vi "In Place Data Modification.vi"() -> ()   [LabVIEW 2019, in "Tree Map.lvlib"]
doc: "<b>Author:</b> Piotr Kruczkowski <PrimaryKey>\n<b>License:</b> NewBSD\n\nCopyright (c) 2019, National Instruments\nAll rights reserved.\n\nRedistribution and use in source and binary forms, with or without\nmodification, are permitted provided that the following conditions are met:\n1. Redistributions of source code must retain the above copyright\n notice, this list of conditions and the following disclaimer.\n2. Redistributions in binary form must reproduce the above copyright\n notice, this list of conditions and the following disclaimer in the\n documentation and/or other materials provided with the distribution.\n3. Neither the name of National Instruments nor the\n names of its contributors may be used to endorse or promote products\n derived from this software without specific prior written permission.\n\nTHIS SOFTWARE IS PROVIDED BY National Instruments ''AS IS'' AND ANY\nEXPRESS OR IMPLIED WARRANTIES, INCLUDING, BUT NOT LIMITED TO, THE IMPLIED\nWARRANTIES OF MERCHANTABILITY AND FITNESS FOR A PARTICULAR PURPOSE ARE\nDISCLAIMED. IN NO EVENT SHALL National Instruments BE LIABLE FOR ANY\nDIRECT, INDIRECT, INCIDENTAL, SPECIAL, EXEMPLARY, OR CONSEQUENTIAL DAMAGES\n(INCLUDING, BUT NOT LIMITED TO, PROCUREMENT OF SUBSTITUTE GOODS OR SERVICES;\nLOSS OF USE, DATA, OR PROFITS; OR BUSINESS INTERRUPTION) HOWEVER CAUSED AND\nON ANY THEORY OF LIABILITY, WHETHER IN CONTRACT, STRICT LIABILITY, OR TORT\n(INCLUDING NEGLIGENCE OR OTHERWISE) ARISING IN ANY WAY OUT OF THE USE OF THIS\nSOFTWARE, EVEN IF ADVISED OF THE POSSIBILITY OF SUCH DAMAGE."
uses:
  Tree Map.lvlib
panel:
  out "Pretty XML":string="<System>\n    <Configuration>\n        <Frequency>50.00</Frequency>\n    </Configuration>\n</System>"
  out "Frequency Node Path":string="\\System\\Configuration\\Frequency"
  in  "New Frequency":dbl=50.0 format="%#_13g"
  in  "Frequency":dbl=123.0 format="%#_13g"
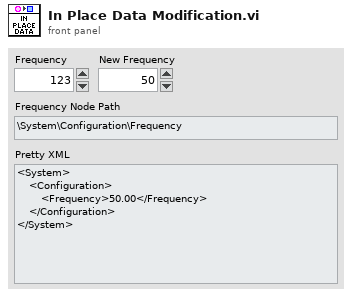
[diagram p1: front panel]
types:
  T1 = typedef "Tree Map.lvlib/Tree Map Data.ctl" = map{string, cluster{"Child Paths Set":set{string}, "Name":string, "Data":string, "Attributes":map{string, string}}}
  T2 = cluster{"Child Paths Set":set{string}, "Name":string, "Data":string, "Attributes":map{string, string}}
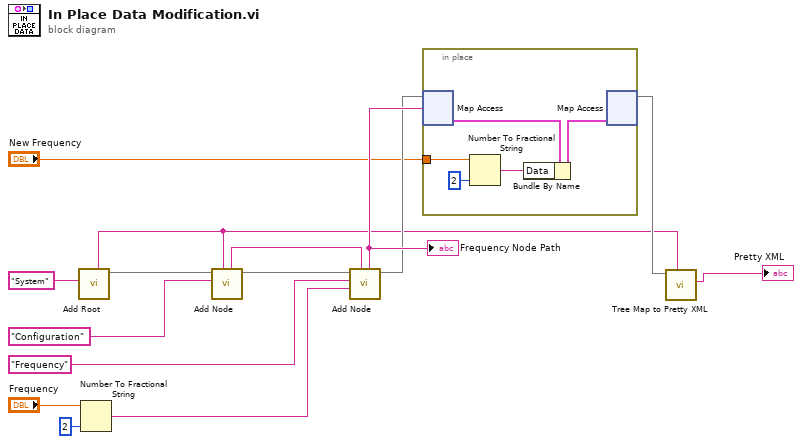
[diagram p0: block diagram]
diagram:
  n1 = call "Add Root.vi"("New Root Name"="System") -> ("Tree Map Out"=w14:T1, "Root Path"=w3:string)  [unwired: 9 in]
  n2 = Number To Fractional String(number="Frequency", precision (6)=i16 2) -> (F-format string=w8:string)  [unwired: 2 in]
  n3 = call "Add Node.vi"("Parent Path"=w3, "New Node Name"="Configuration", "Tree Map In"=w14) -> ("Tree Map Out"=w11:T1, "New Node Path"=w12:string)  [unwired: 6 in, 1 out]
  n4 = call "Add Node.vi"("Parent Path"=w12, "Data"=w8, "New Node Name"="Frequency", "Tree Map In"=w11) -> ("Tree Map Out"=w6:T1, "New Node Path"=w7:string)  [unwired: 5 in, 1 out]
  "Frequency Node Path" <- w7
  n5 = in-place {
    in-place-border: "New Frequency" -> [w17]
    n6 = in-place-map #1(w6, w7) -> (w20:T2)  [unwired: 1 in, 1 out]
    n7 = Number To Fractional String(number=w17, precision (6)=i16 2) -> (F-format string=w18:string)  [unwired: 2 in]
    n8 = Bundle By Name(cluster=w20, "Data"=w18) -> (w19:T2)
    n9 = in-place-map #1(w19) -> (w5:T1)  [unwired: 1 in, 2 out]
  }
  n10 = call "Tree Map to Pretty XML.vi"("Root Path"=w3, "Tree Map In"=w5) -> ("Pretty XML"=→"Pretty XML":string)  [unwired: 8 in, 1 out]
